vi "初始化注册表.vi"(8 "error in (no error)":errorcluster caption="错误输入（无错误）") -> (0 "error out":errorcluster caption="错误输出")   [LabVIEW 2014]
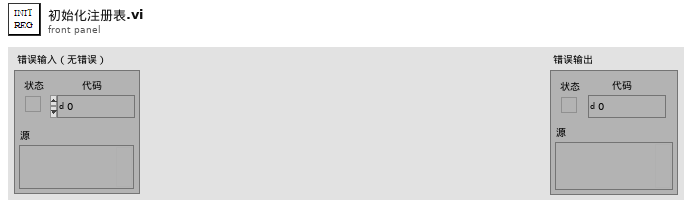
[diagram p1: front panel]
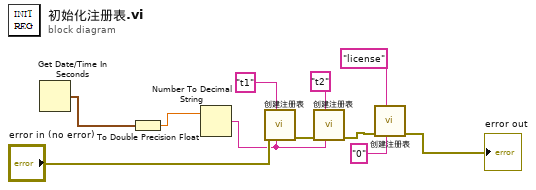
[diagram p0: block diagram]
diagram:
  n1 = Get Date/Time In Seconds() -> (seconds since 1Jan1904=w5:timestamp)
  n2 = To Double Precision Float(number=w5) -> (double precision float=w11:dbl)
  n3 = Number To Decimal String(number=w11) -> (decimal integer string=w6:string)  [unwired: 1 in]
  n4 = call "创建注册表.vi"("写入内容"=w6, "键名称"="t1", "error in (no error)"="error in (no error)") -> ("error out"=w9:errorcluster)  [unwired: 8 in]
  n5 = call "创建注册表.vi"("写入内容"=w6, "键名称"="t2", "error in (no error)"=w9) -> ("error out"=w4:errorcluster)  [unwired: 8 in]
  n6 = call "创建注册表.vi"("写入内容"="0", "键名称"="license", "error in (no error)"=w4) -> ("error out"=→"error out":errorcluster)  [unwired: 8 in]
